vi "xps_get_stored_trajectory_names.vi"(8 "error in (no error)":errorcluster, 11 "newport_xps in":refnum<class "newport_xps.lvclass">) -> (0 "error out":errorcluster, 2 "trajectory_names":string[](array[string]), 3 "newport_xps out":refnum<class "newport_xps.lvclass">)   [LabVIEW 2015, in "newport_xps.lvclass"]
uses:
  newport_xps.lvclass
  newport_xps.lvclass/newport_xps.ctl
  <vilib>/FTP/NI_FTP.lvlib
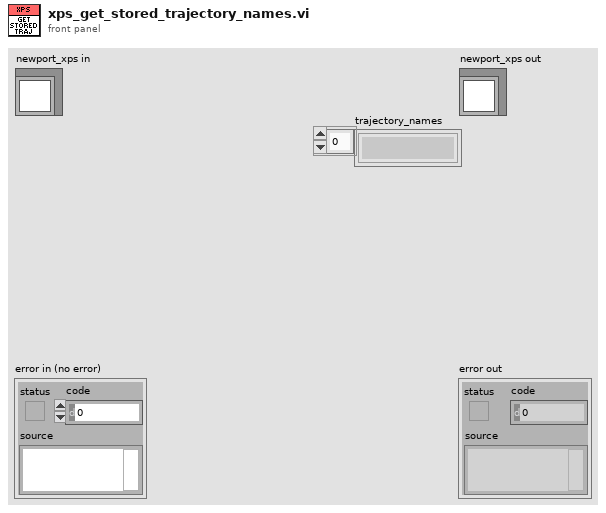
[diagram p1: front panel]
types:
  T1 = typedef "NI_FTP.lvlib/FTP Session.ctl" = refnum<k5>
  T2 = typedef "NI_FTP.lvlib/FTP File Info.ctl" = cluster{"type":enum16{"unknown", "file", "dir", "link"}, "permissions":string, "owner":string, "group":string, "size":i32, "date":string, "name":string, "link name":string}
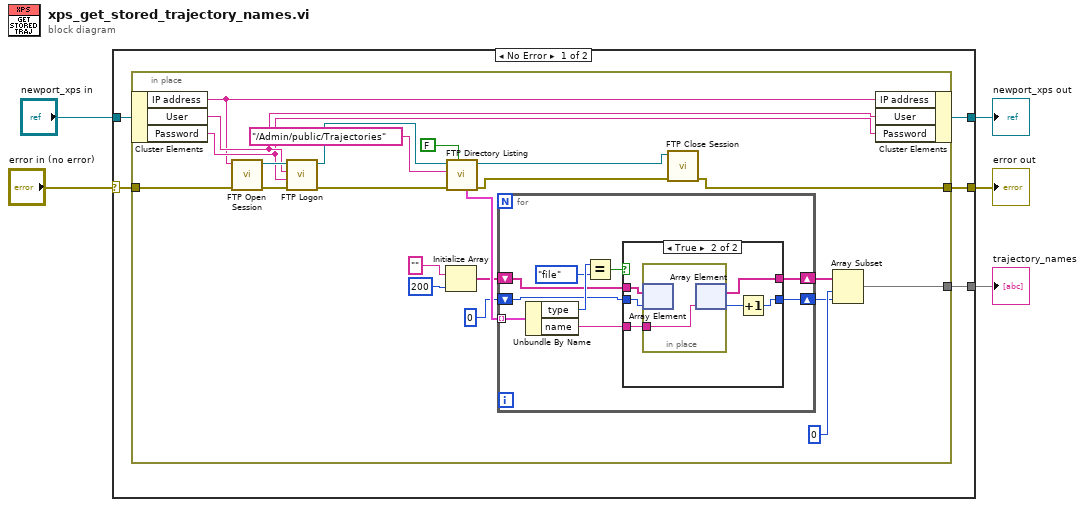
[diagram p0: block diagram]
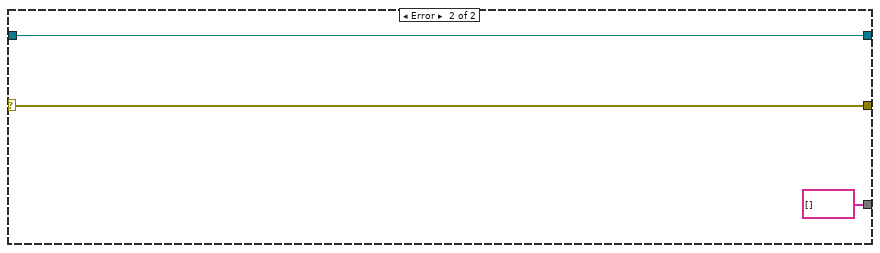
[diagram p3: hidden frame]
diagram:
  n1 = case shown="No Error" "error in (no error)" {
    selector: "error in (no error)" -> [w9 w53]
    tunnel: [w6 w53] -> w4
    tunnel: [w7 w52] -> w2
    tunnel: "newport_xps in" -> [w10 w52]
    tunnel: [w8 string[] []] -> w1
    frame No Error {
      n2 = in-place {
        in-place-border: w9 -> [w25]
        in-place-border: [w14] -> w8
        in-place-border: [w11] -> w6
        n3 = in-place-cluster #1(w10) -> ("IP address"=w29:string, "User"=w31:string, "Password"=w30:string)
        n4 = call <vilib>:"FTP Open Session.vi"("error in (no error)"=w25, "address"=w29) -> ("error out"=w26:errorcluster, "ftp session"=w32:T1)  [unwired: 6 in, 2 out]
        n5 = call <vilib>:"FTP Logon.vi"("error in (no error)"=w26, "password"=w30, "user"=w31, "ftp session"=w32) -> ("error out"=w27:errorcluster, "ftp session out"=w24:T1)  [unwired: 4 in, 2 out]
        n6 = Initialize Array("", 200 ("dimension size")) -> (w19:string[])
        n7 = call <vilib>:"FTP Directory Listing.vi"("active (T)"=FALSE, "error in (no error)"=w27, "directory path"="/Admin/public/Trajectories", "ftp session"=w24) -> ("error out"=w13:errorcluster, "ftp session out"=w12:T1, "dir list"=w20:T2[])  [unwired: 3 in, 2 out]
        n8 = for {
          tunnel: w20 -> [w41] mode=indexing
          shift-right: [w33] -> w17
          shift-left: w19 -> [w38]
          shift-right: [w34] -> w15
          shift-left: 0 -> [w37]
          n9 = Unbundle By Name(w41) -> ("type"=w40:enum16{"unknown", "file", "dir", "link"}, "name"=w35:string)
          n10 = Equal?(x=w40, y=enum16{"unknown", "file", "dir", "link"}."file") -> (x = y?=w36:bool)
          n11 = case shown="True" w36 {
            tunnel: w38 -> [w43 w49]
            tunnel: w37 -> [w42 w48]
            tunnel: w35 -> [_ w47]
            tunnel: [w42 w45] -> w34
            tunnel: [w43 w44] -> w33
            frame False {
            }
            frame True {
              n12 = in-place {
                in-place-border: w47 -> [w50]
                n13 = in-place-array #2(w49, w48) -> ()  [unwired: 1 out]
                n14 = in-place-array #2(w50) -> (w44:string[], w46:i32)
              }
              n15 = Increment(x=w46) -> (x+1=w45:i32)
            }
          }
        }
        n16 = call <vilib>:"FTP Close Session.vi"("error in (no error)"=w13, "ftp session"=w12) -> ("error out"=w11:errorcluster)  [unwired: 6 in, 3 out]
        n17 = Array Subset(array=w17, index=0, length=w15) -> (w14:string[])
        n18 = in-place-cluster #1("IP address"=w29, "User"=w31, "Password"=w30) -> (w7:refnum<class "newport_xps.lvclass">)
      }
    }
    frame Error {
    }
  }
  "error out" <- w4
  "newport_xps out" <- w2
  "trajectory_names" <- w1
